vi "test-Coordinate-System-Test6.vi"() -> (3 "All tests passed":bool)   [LabVIEW 2019]
uses:
  <vilib>/Rock Robotics/WPI/ThirdParty/JAS_Junk/TrajLib/VI/CoordAxis_N.vi
  <vilib>/Rock Robotics/WPI/ThirdParty/JAS_Junk/TrajLib/VI/CoordSystem_New.vi
  <vilib>/Rock Robotics/WPI/ThirdParty/JAS_Junk/TrajLib/VI/CoordAxis_E.vi
  <vilib>/Rock Robotics/WPI/ThirdParty/JAS_Junk/TrajLib/VI/CoordAxis_D.vi
  <vilib>/Rock Robotics/WPI/ThirdParty/JAS_Junk/TrajLib/Conv_Deg_Radians.vi
  <vilib>/Rock Robotics/WPI/ThirdParty/JAS_Junk/TrajLib/VI/Quaternion_New.vi
  <vilib>/Rock Robotics/WPI/ThirdParty/JAS_Junk/TrajLib/VI/CoordAxis_New.vi
  <vilib>/Rock Robotics/WPI/ThirdParty/JAS_Junk/TrajLib/MatBuilder_Create.vi
  <vilib>/Rock Robotics/WPI/ThirdParty/JAS_Junk/TrajLib/Matrix_AssignBlock.vi
  <vilib>/Rock Robotics/WPI/ThirdParty/JAS_Junk/TrajLib/VI/Rotation3D_Create_RotMatrix.vi
  <vilib>/Rock Robotics/WPI/ThirdParty/JAS_Junk/TrajLib/MatrixHelper_CoerceSize.vi
  <vilib>/Rock Robotics/WPI/ThirdParty/JAS_Junk/TrajLib/VI/Rotation3d_Create_Quaternion.vi
  <vilib>/Rock Robotics/WPI/ThirdParty/JAS_Junk/TrajLib/Matrix_Transpose.vi
  <vilib>/Analysis/baseanly.llb/A x B.vi
  <vilib>/Analysis/baseanly.llb/Real A x B.vi
  <vilib>/Rock Robotics/WPI/ThirdParty/JAS_Junk/TrajLib/Matrix_Ident.vi
  <vilib>/Rock Robotics/WPI/ThirdParty/JAS_Junk/TrajLib/Matrix_IsEqual.vi
  <vilib>/Analysis/baseanly.llb/Determinant.vi
  <vilib>/Analysis/baseanly.llb/Real Determinant.vi
  <vilib>/Rock Robotics/WPI/ThirdParty/JAS_Junk/TrajLib/VI/Quaternion_Normalize.vi
  <vilib>/Rock Robotics/WPI/ThirdParty/JAS_Junk/TrajLib/VI/Quaternion_New_Default.vi
  <vilib>/Analysis/Matrix/Numeric/Conversions/Array To Matrix.vi
  <vilib>/Analysis/Matrix/Numeric/Conversions/Array To Matrix - RA.vi
  <vilib>/Analysis/7linalg.llb/Create Special Matrix.vi
  <vilib>/Analysis/7linalg.llb/Create Special Real Matrix.vi
  <vilib>/Rock Robotics/WPI/ThirdParty/JAS_Junk/TrajLib/Trajectory_Library.lvlib
panel:
  out "Test 4":bool
  out "Test 3":bool
  out "Test 2":bool
  out "Test 1":bool
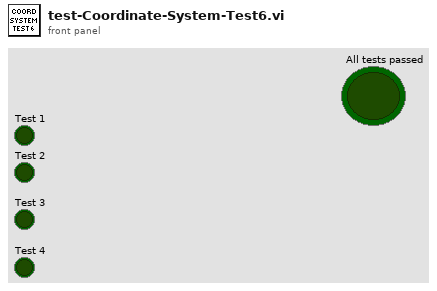
[diagram p1: front panel]
types:
  T1 = typedef "Trajectory_Library.lvlib/TRANSLATION3D.ctl" = cluster{"X":dbl, "Y":dbl, "Z":dbl}
  T2 = typedef "Trajectory_Library.lvlib/ROTATION3D.ctl" = cluster{"Q_quaternion":T3}
  T3 = typedef "Trajectory_Library.lvlib/QUATERNION.ctl" = cluster{"R":dbl, "V":dbl[]}
  T4 = typedef "Trajectory_Library.lvlib/TRANSFORM3D.ctl" = cluster{"TRANSLATION3D":T1, "ROTATION3D":T2, "XF":bool}
  T5 = typedef "Trajectory_Library.lvlib/COORDINATE_SYSTEM.ctl" = cluster{"Rotation":T2}
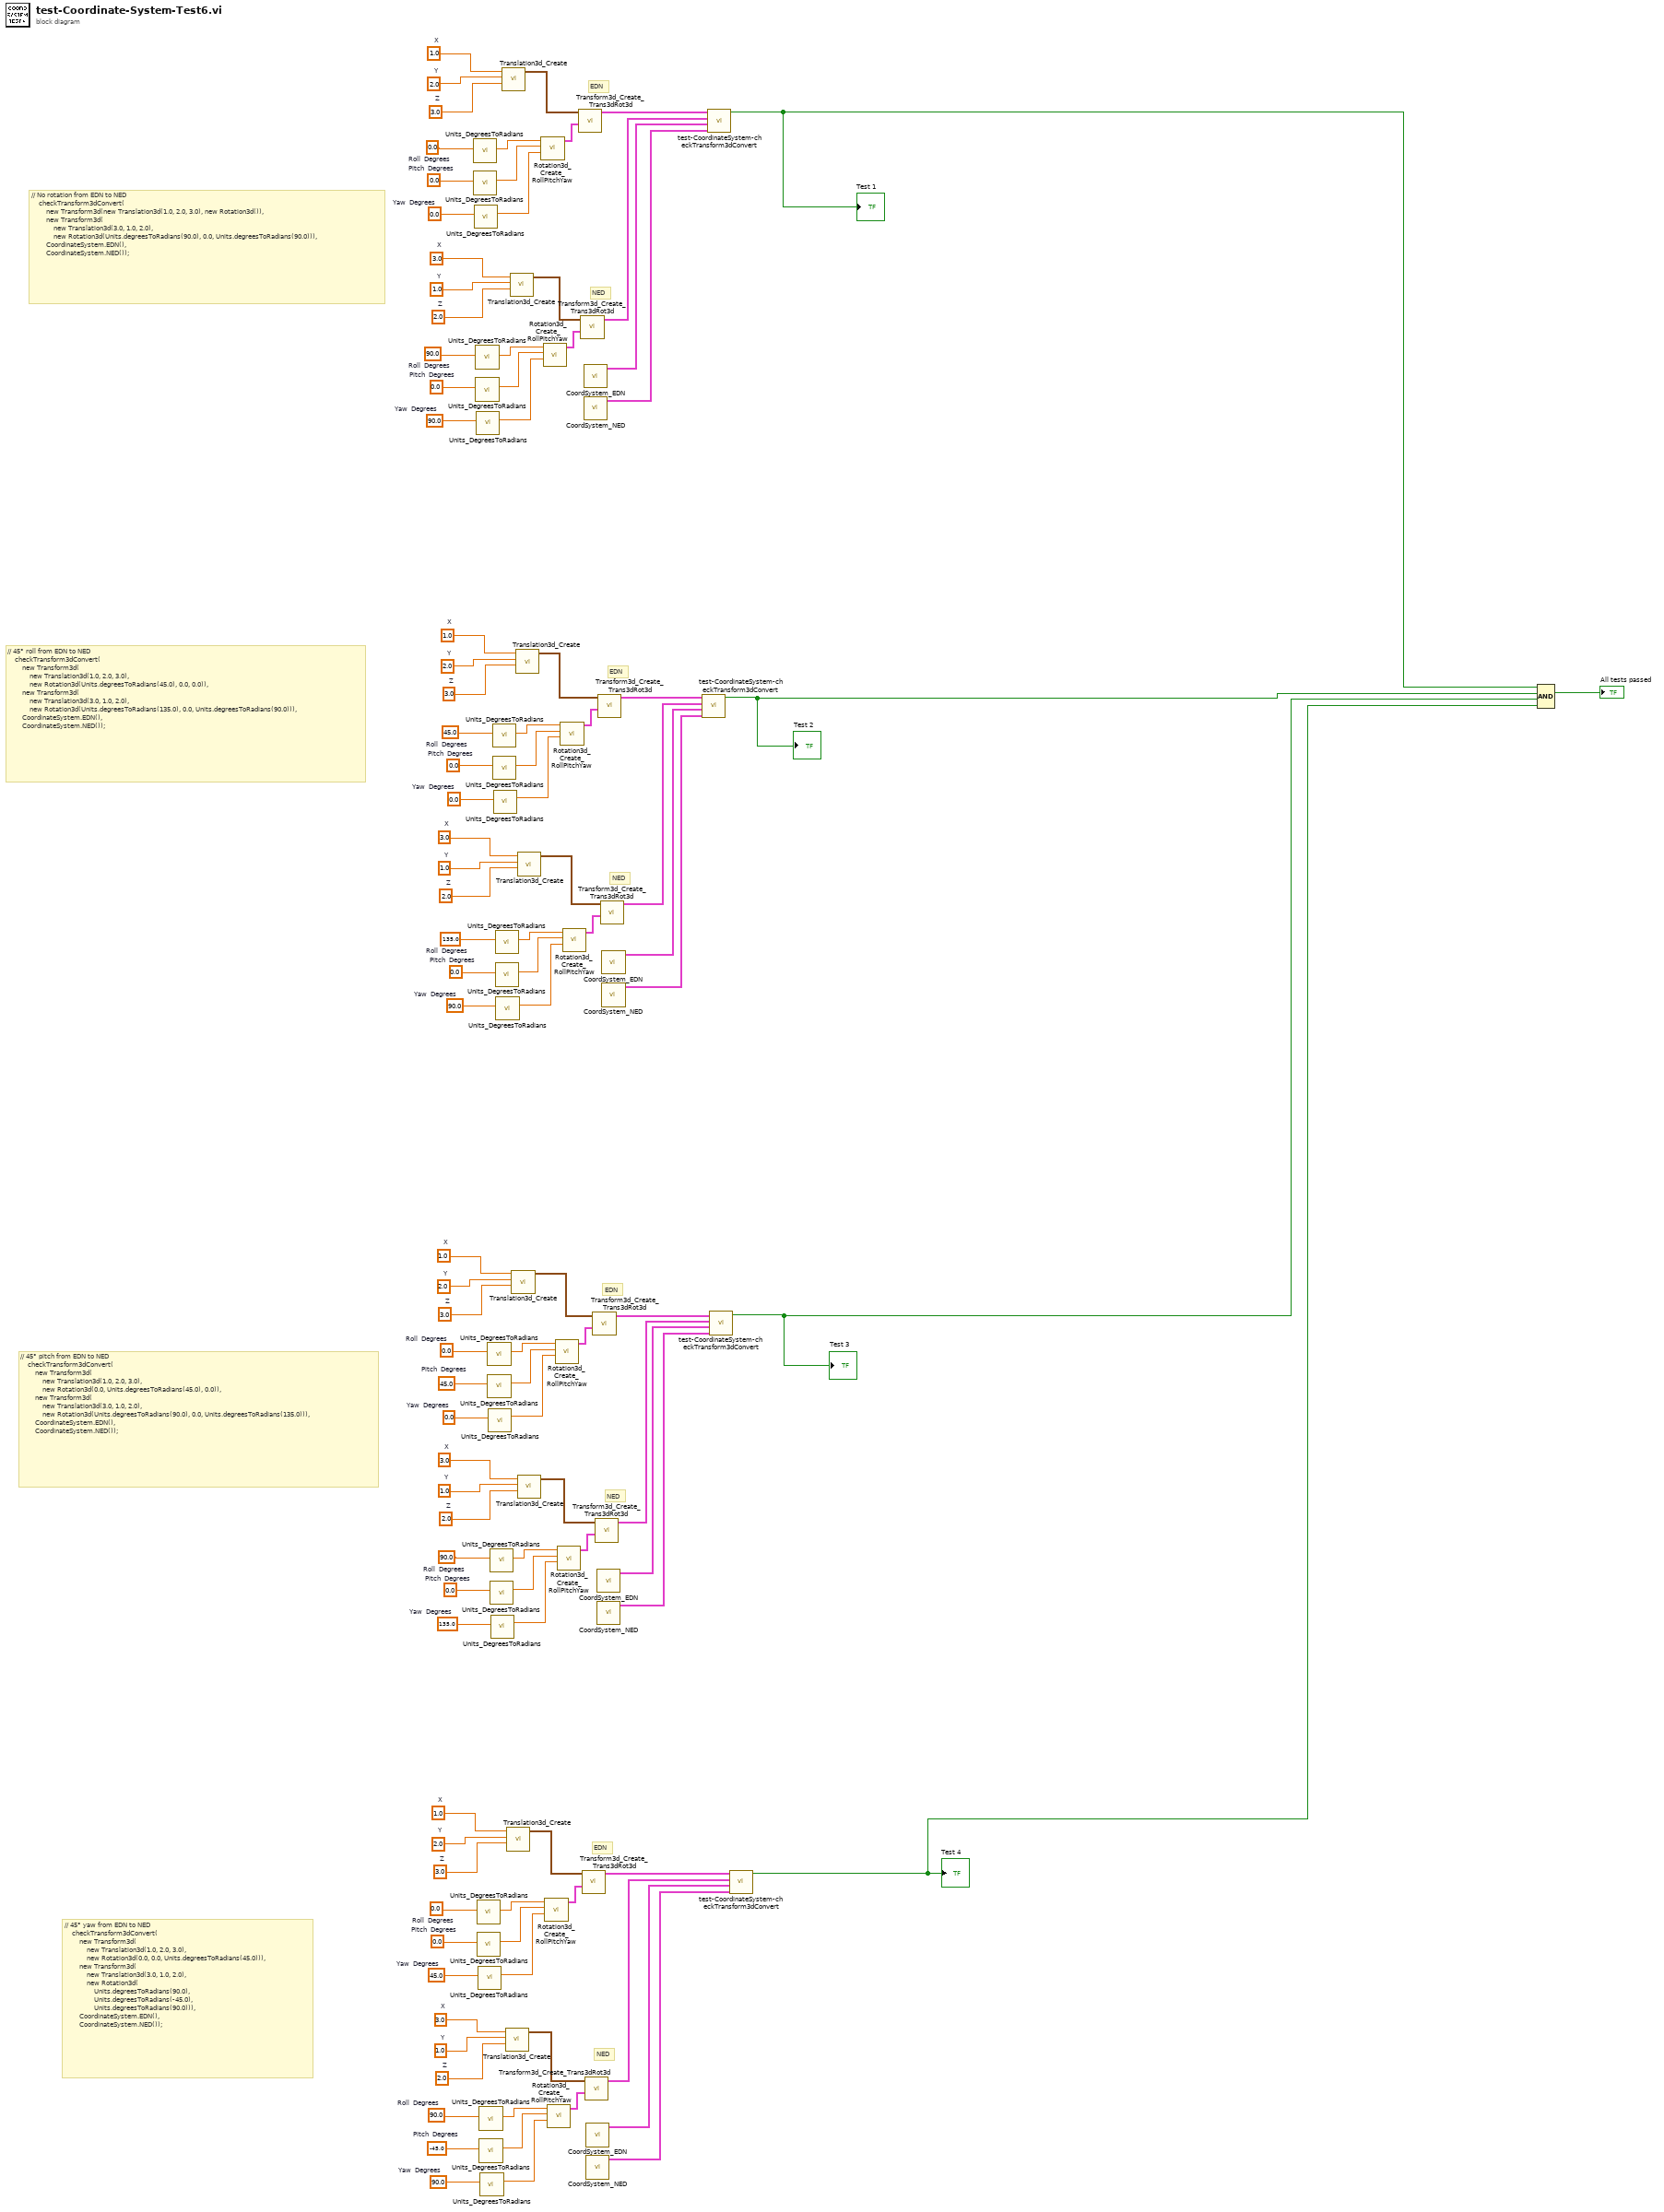
[diagram p0: block diagram]
diagram:
  w5 = 3.0  # X
  w4 = 1.0  # Y
  w3 = 2.0  # Z
  w9 = 3.0  # X
  w8 = 1.0  # Y
  w7 = 2.0  # Z
  w17 = 1.0  # X
  w16 = 2.0  # Y
  w15 = 3.0  # Z
  w21 = 1.0  # X
  w20 = 2.0  # Y
  w19 = 3.0  # Z
  w25 = 1.0  # X
  w24 = 2.0  # Y
  w23 = 3.0  # Z
  w29 = 3.0  # X
  w28 = 1.0  # Y
  w27 = 2.0  # Z
  w53 = 90.0  # Roll  Degrees
  w54 = -45.0  # Pitch  Degrees
  w55 = 90.0  # Yaw  Degrees
  w32 = 1.0  # X
  w31 = 2.0  # Y
  w30 = 3.0  # Z
  w60 = 0.0  # Roll  Degrees
  w61 = 0.0  # Pitch  Degrees
  w62 = 45.0  # Yaw  Degrees
  w67 = 90.0  # Roll  Degrees
  w68 = 0.0  # Pitch  Degrees
  w69 = 135.0  # Yaw  Degrees
  w74 = 0.0  # Roll  Degrees
  w75 = 45.0  # Pitch  Degrees
  w76 = 0.0  # Yaw  Degrees
  w81 = 135.0  # Roll  Degrees
  w82 = 0.0  # Pitch  Degrees
  w83 = 90.0  # Yaw  Degrees
  w88 = 45.0  # Roll  Degrees
  w89 = 0.0  # Pitch  Degrees
  w90 = 0.0  # Yaw  Degrees
  w13 = 3.0  # X
  w12 = 1.0  # Y
  w11 = 2.0  # Z
  w96 = 90.0  # Roll  Degrees
  w97 = 0.0  # Pitch  Degrees
  w98 = 90.0  # Yaw  Degrees
  w103 = 0.0  # Roll  Degrees
  w104 = 0.0  # Pitch  Degrees
  w105 = 0.0  # Yaw  Degrees
  # "// 45° pitch from EDN to NED\n    checkTransform3dConvert(\n        new Transform3d(\n            new Translation3d(1.0, 2.0, 3.0),\n            new Rotation3d(0.0, Units.degreesToRadians(45.0), 0.0)),\n        new Transform3d(\n            new Translation3d(3.0, 1.0, 2.0),\n            new Rotation3d(Units.degreesToRadians(90.0), 0.0, Units.degreesToRadians(135.0))),\n        CoordinateSystem.EDN(),\n        CoordinateSystem.NED());"
  # "// 45° roll from EDN to NED\n    checkTransform3dConvert(\n        new Transform3d(\n            new Translation3d(1.0, 2.0, 3.0),\n            new Rotation3d(Units.degreesToRadians(45.0), 0.0, 0.0)),\n        new Transform3d(\n            new Translation3d(3.0, 1.0, 2.0),\n            new Rotation3d(Units.degreesToRadians(135.0), 0.0, Units.degreesToRadians(90.0))),\n        CoordinateSystem.EDN(),\n        CoordinateSystem.NED());"
  # "// No rotation from EDN to NED\n    checkTransform3dConvert(\n        new Transform3d(new Translation3d(1.0, 2.0, 3.0), new Rotation3d()),\n        new Transform3d(\n            new Translation3d(3.0, 1.0, 2.0),\n            new Rotation3d(Units.degreesToRadians(90.0), 0.0, Units.degreesToRadians(90.0))),\n        CoordinateSystem.EDN(),\n        CoordinateSystem.NED());"
  # "// 45° yaw from EDN to NED\n    checkTransform3dConvert(\n        new Transform3d(\n            new Translation3d(1.0, 2.0, 3.0),\n            new Rotation3d(0.0, 0.0, Units.degreesToRadians(45.0))),\n        new Transform3d(\n            new Translation3d(3.0, 1.0, 2.0),\n            new Rotation3d(\n                Units.degreesToRadians(90.0),\n                Units.degreesToRadians(-45.0),\n                Units.degreesToRadians(90.0))),\n        CoordinateSystem.EDN(),\n        CoordinateSystem.NED());"
  # "NED"
  # "EDN"
  # "NED"
  # "EDN"
  # "NED"
  # "EDN"
  # "NED"
  # "EDN"
  n1 = call <vilib>:"Units_DegreesToRadians.vi"("Degrees"=w103) -> ("Radians"=w106:dbl)  [unwired: 10 in]
  n2 = call <vilib>:"Units_DegreesToRadians.vi"("Degrees"=w104) -> ("Radians"=w107:dbl)  [unwired: 10 in]
  n3 = call <vilib>:"Units_DegreesToRadians.vi"("Degrees"=w105) -> ("Radians"=w108:dbl)  [unwired: 10 in]
  n4 = call <vilib>:"Units_DegreesToRadians.vi"("Degrees"=w96) -> ("Radians"=w99:dbl)  [unwired: 10 in]
  n5 = call <vilib>:"Units_DegreesToRadians.vi"("Degrees"=w97) -> ("Radians"=w100:dbl)  [unwired: 10 in]
  n6 = call <vilib>:"Units_DegreesToRadians.vi"("Degrees"=w98) -> ("Radians"=w101:dbl)  [unwired: 10 in]
  n7 = call <vilib>:"Units_DegreesToRadians.vi"("Degrees"=w60) -> ("Radians"=w63:dbl)  [unwired: 10 in]
  n8 = call <vilib>:"Units_DegreesToRadians.vi"("Degrees"=w61) -> ("Radians"=w64:dbl)  [unwired: 10 in]
  n9 = call <vilib>:"Units_DegreesToRadians.vi"("Degrees"=w62) -> ("Radians"=w65:dbl)  [unwired: 10 in]
  n10 = call <vilib>:"Units_DegreesToRadians.vi"("Degrees"=w53) -> ("Radians"=w56:dbl)  [unwired: 10 in]
  n11 = call <vilib>:"Units_DegreesToRadians.vi"("Degrees"=w54) -> ("Radians"=w57:dbl)  [unwired: 10 in]
  n12 = call <vilib>:"Units_DegreesToRadians.vi"("Degrees"=w55) -> ("Radians"=w58:dbl)  [unwired: 10 in]
  n13 = call <vilib>:"Units_DegreesToRadians.vi"("Degrees"=w74) -> ("Radians"=w77:dbl)  [unwired: 10 in]
  n14 = call <vilib>:"Units_DegreesToRadians.vi"("Degrees"=w75) -> ("Radians"=w78:dbl)  [unwired: 10 in]
  n15 = call <vilib>:"Units_DegreesToRadians.vi"("Degrees"=w76) -> ("Radians"=w79:dbl)  [unwired: 10 in]
  n16 = call <vilib>:"Units_DegreesToRadians.vi"("Degrees"=w67) -> ("Radians"=w70:dbl)  [unwired: 10 in]
  n17 = call <vilib>:"Units_DegreesToRadians.vi"("Degrees"=w68) -> ("Radians"=w71:dbl)  [unwired: 10 in]
  n18 = call <vilib>:"Units_DegreesToRadians.vi"("Degrees"=w69) -> ("Radians"=w72:dbl)  [unwired: 10 in]
  n19 = call <vilib>:"Units_DegreesToRadians.vi"("Degrees"=w88) -> ("Radians"=w91:dbl)  [unwired: 10 in]
  n20 = call <vilib>:"Units_DegreesToRadians.vi"("Degrees"=w89) -> ("Radians"=w92:dbl)  [unwired: 10 in]
  n21 = call <vilib>:"Units_DegreesToRadians.vi"("Degrees"=w90) -> ("Radians"=w93:dbl)  [unwired: 10 in]
  n22 = call <vilib>:"Units_DegreesToRadians.vi"("Degrees"=w81) -> ("Radians"=w84:dbl)  [unwired: 10 in]
  n23 = call <vilib>:"Units_DegreesToRadians.vi"("Degrees"=w82) -> ("Radians"=w85:dbl)  [unwired: 10 in]
  n24 = call <vilib>:"Units_DegreesToRadians.vi"("Degrees"=w83) -> ("Radians"=w86:dbl)  [unwired: 10 in]
  n25 = call <vilib>:"Translation3d_Create.vi"("Z"=w15, "Y"=w16, "X"=w17) -> ("TRANSLATION3D"=w14:T1)  [unwired: 8 in]
  n26 = call <vilib>:"Translation3d_Create.vi"("Z"=w27, "Y"=w28, "X"=w29) -> ("TRANSLATION3D"=w1:T1)  [unwired: 8 in]
  n27 = call <vilib>:"Translation3d_Create.vi"("Z"=w30, "Y"=w31, "X"=w32) -> ("TRANSLATION3D"=w26:T1)  [unwired: 8 in]
  n28 = call <vilib>:"Translation3d_Create.vi"("Z"=w11, "Y"=w12, "X"=w13) -> ("TRANSLATION3D"=w10:T1)  [unwired: 8 in]
  n29 = call <vilib>:"Translation3d_Create.vi"("Z"=w23, "Y"=w24, "X"=w25) -> ("TRANSLATION3D"=w22:T1)  [unwired: 8 in]
  n30 = call <vilib>:"Translation3d_Create.vi"("Z"=w19, "Y"=w20, "X"=w21) -> ("TRANSLATION3D"=w18:T1)  [unwired: 8 in]
  n31 = call <vilib>:"Translation3d_Create.vi"("Z"=w7, "Y"=w8, "X"=w9) -> ("TRANSLATION3D"=w6:T1)  [unwired: 8 in]
  n32 = call <vilib>:"Translation3d_Create.vi"("Z"=w3, "Y"=w4, "X"=w5) -> ("TRANSLATION3D"=w2:T1)  [unwired: 8 in]
  n33 = call <vilib>:"Rotation3d_Create_RollPitchYaw.vi"("Yaw"=w108, "Pitch"=w107, "Roll"=w106) -> ("Rotation3d"=w109:T2)  [unwired: 8 in]
  n34 = call <vilib>:"Rotation3d_Create_RollPitchYaw.vi"("Yaw"=w101, "Pitch"=w100, "Roll"=w99) -> ("Rotation3d"=w102:T2)  [unwired: 8 in]
  n35 = call <vilib>:"Rotation3d_Create_RollPitchYaw.vi"("Yaw"=w65, "Pitch"=w64, "Roll"=w63) -> ("Rotation3d"=w66:T2)  [unwired: 8 in]
  n36 = call <vilib>:"Rotation3d_Create_RollPitchYaw.vi"("Yaw"=w58, "Pitch"=w57, "Roll"=w56) -> ("Rotation3d"=w59:T2)  [unwired: 8 in]
  n37 = call <vilib>:"Rotation3d_Create_RollPitchYaw.vi"("Yaw"=w79, "Pitch"=w78, "Roll"=w77) -> ("Rotation3d"=w80:T2)  [unwired: 8 in]
  n38 = call <vilib>:"Rotation3d_Create_RollPitchYaw.vi"("Yaw"=w72, "Pitch"=w71, "Roll"=w70) -> ("Rotation3d"=w73:T2)  [unwired: 8 in]
  n39 = call <vilib>:"Rotation3d_Create_RollPitchYaw.vi"("Yaw"=w93, "Pitch"=w92, "Roll"=w91) -> ("Rotation3d"=w94:T2)  [unwired: 8 in]
  n40 = call <vilib>:"Rotation3d_Create_RollPitchYaw.vi"("Yaw"=w86, "Pitch"=w85, "Roll"=w84) -> ("Rotation3d"=w87:T2)  [unwired: 8 in]
  n41 = call <vilib>:"Transform3d_Create_Trans3dRot3d.vi"("Rotation3d"=w109, "Translation3d"=w14) -> ("Transform3d"=w37:T4)  [unwired: 9 in]
  n42 = call <vilib>:"Transform3d_Create_Trans3dRot3d.vi"("Rotation3d"=w102, "Translation3d"=w10) -> ("Transform3d"=w36:T4)  [unwired: 9 in]
  n43 = call <vilib>:"Transform3d_Create_Trans3dRot3d.vi"("Rotation3d"=w66, "Translation3d"=w26) -> ("Transform3d"=w52:T4)  [unwired: 9 in]
  n44 = call <vilib>:"CoordSystem_EDN.vi"() -> ("out Coordinate System"=w35:T5)  [unwired: 10 in, 1 out]
  n45 = call <vilib>:"CoordSystem_NED.vi"() -> ("out Coordinate System"=w34:T5)  [unwired: 10 in, 1 out]
  n46 = call <vilib>:"Transform3d_Create_Trans3dRot3d.vi"("Rotation3d"=w59, "Translation3d"=w1) -> ("Transform3d"=w51:T4)  [unwired: 9 in]
  n47 = call <vilib>:"CoordSystem_EDN.vi"() -> ("out Coordinate System"=w50:T5)  [unwired: 10 in, 1 out]
  n48 = call <vilib>:"CoordSystem_NED.vi"() -> ("out Coordinate System"=w49:T5)  [unwired: 10 in, 1 out]
  n49 = call <vilib>:"Transform3d_Create_Trans3dRot3d.vi"("Rotation3d"=w80, "Translation3d"=w22) -> ("Transform3d"=w47:T4)  [unwired: 9 in]
  n50 = call <vilib>:"Transform3d_Create_Trans3dRot3d.vi"("Rotation3d"=w73, "Translation3d"=w2) -> ("Transform3d"=w46:T4)  [unwired: 9 in]
  n51 = call <vilib>:"CoordSystem_EDN.vi"() -> ("out Coordinate System"=w44:T5)  [unwired: 10 in, 1 out]
  n52 = call <vilib>:"CoordSystem_NED.vi"() -> ("out Coordinate System"=w45:T5)  [unwired: 10 in, 1 out]
  n53 = call <vilib>:"Transform3d_Create_Trans3dRot3d.vi"("Rotation3d"=w94, "Translation3d"=w18) -> ("Transform3d"=w42:T4)  [unwired: 9 in]
  n54 = call <vilib>:"Transform3d_Create_Trans3dRot3d.vi"("Rotation3d"=w87, "Translation3d"=w6) -> ("Transform3d"=w41:T4)  [unwired: 9 in]
  n55 = call <vilib>:"CoordSystem_EDN.vi"() -> ("out Coordinate System"=w40:T5)  [unwired: 10 in, 1 out]
  n56 = call <vilib>:"CoordSystem_NED.vi"() -> ("out Coordinate System"=w39:T5)  [unwired: 10 in, 1 out]
  n57 = call "test-CoordinateSystem-checkTransform3dConvert.vi"("COORDINATE_SYSTEM_TO"=w39, "COORDINATE_SYSTEM_FROM"=w40, "Transform3D_TO"=w41, "Transform3D_FROM"=w42) -> ("All tests passed"=w38:bool)  [unwired: 7 in]
  "Test 2" <- w38
  n58 = call "test-CoordinateSystem-checkTransform3dConvert.vi"("COORDINATE_SYSTEM_TO"=w34, "COORDINATE_SYSTEM_FROM"=w35, "Transform3D_TO"=w36, "Transform3D_FROM"=w37) -> ("All tests passed"=w33:bool)  [unwired: 7 in]
  "Test 1" <- w33
  n59 = call "test-CoordinateSystem-checkTransform3dConvert.vi"("COORDINATE_SYSTEM_TO"=w45, "COORDINATE_SYSTEM_FROM"=w44, "Transform3D_TO"=w46, "Transform3D_FROM"=w47) -> ("All tests passed"=w43:bool)  [unwired: 7 in]
  "Test 3" <- w43
  n60 = call "test-CoordinateSystem-checkTransform3dConvert.vi"("COORDINATE_SYSTEM_TO"=w49, "COORDINATE_SYSTEM_FROM"=w50, "Transform3D_TO"=w51, "Transform3D_FROM"=w52) -> ("All tests passed"=w48:bool)  [unwired: 7 in]
  "Test 4" <- w48
  n61 = Compound Arithmetic op=AND(w33, w38, w43, w48) -> (→"All tests passed":bool)
